vi "Read Number of Tatics.vi"(8 "error in (no error)":errorcluster, 11 "SimplePassRollRole in":refnum<class "SimplePassRollRole.lvclass">) -> (0 "error out":errorcluster, 2 "Number of Tatics":dbl, 3 "SimplePassRollRole out":refnum<class "SimplePassRollRole.lvclass">)   [LabVIEW 2023, in "SimplePassRollRole.lvclass"]
uses:
  SimplePassRollRole.lvclass
  SimplePassRollRole.lvclass/SimplePassRollRole.ctl
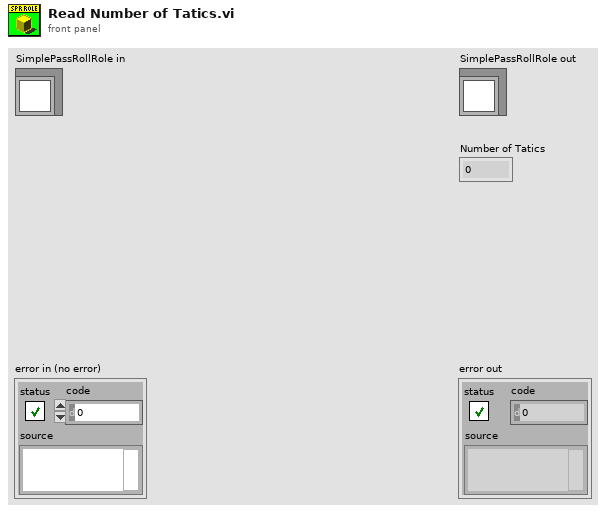
[diagram p1: front panel]
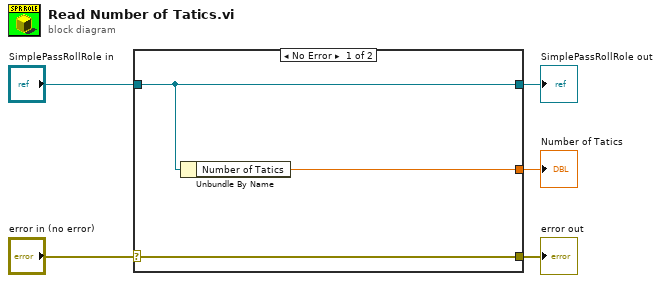
[diagram p0: block diagram]
diagram:
  n1 = case shown="No Error" "error in (no error)" {
    selector: "error in (no error)" -> [w8 w9]
    tunnel: [w8 w9] -> w4
    tunnel: [w7 w10] -> w2
    tunnel: "SimplePassRollRole in" -> [w7 w10]
    tunnel: [w6 _] -> w1
    frame No Error {
      n2 = Unbundle By Name(w7) -> ("Number of Tatics"=w6:dbl)
    }
    frame Error {
    }
  }
  "error out" <- w4
  "SimplePassRollRole out" <- w2
  "Number of Tatics" <- w1
